vi "RunOnce.vi"(1 "Mode":enum16{"Reset", "Run"}(ring)) -> (0 "State":enum16{"RunOnce", "Finished"}(ring))   [LabVIEW 2011]
panel:
  out "InternalState":enum16{"RunOnce", "Finished"}(ring)
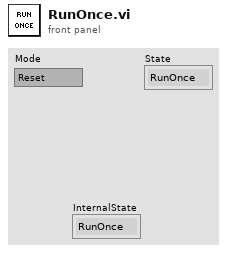
[diagram p1: front panel]
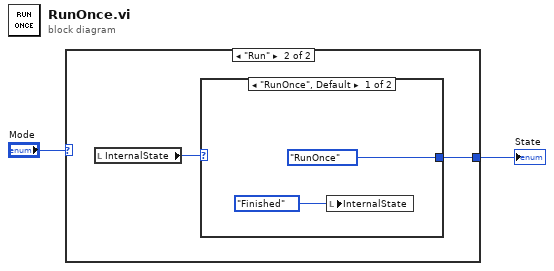
[diagram p0: block diagram]
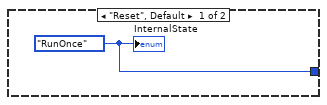
[diagram p2: hidden frame]
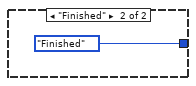
[diagram p3: hidden frame]
diagram:
  n1 = case shown="\"Run\"" "Mode" {
    tunnel: [w3 w4] -> w1
    frame "Reset", Default {
      w3 = enum16{"RunOnce", "Finished"}."RunOnce" ("State")
      "InternalState" <- w3
    }
    frame "Run" {
      n2 = local read "InternalState"() -> (w5:enum16{"RunOnce", "Finished"})
      n3 = case shown="\"RunOnce\", Default" w5 {
        tunnel: [enum16{"RunOnce", "Finished"}."RunOnce" ("State") enum16{"RunOnce", "Finished"}."Finished" ("State")] -> w4
        frame "RunOnce", Default {
          n4 = local write "InternalState"(enum16{"RunOnce", "Finished"}."Finished" ("State")) -> ()
        }
        frame "Finished" {
        }
      }
    }
  }
  "State" <- w1
